vi "Avocent_build_command_OFF.vi"(8 "error in":errorcluster, 11 "Set switches":bool[](array[boolean])=[FALSE, TRUE, TRUE, FALSE, TRUE, TRUE, FALSE, FALSE, TRUE, FALSE, TRUE, TRUE, TRUE, TRUE, TRUE, TRUE, FALSE, FALSE, FALSE, FALSE, FALSE, FALSE, FALSE, FALSE, FALSE, FALSE, FALSE, FALSE, FALSE, FALSE, FALSE, FALSE] caption="Set Switches") -> (0 "error out":errorcluster, 3 "HTTP command":string="/3?3=admin,1234,1001001101000000,")   [LabVIEW 2013]
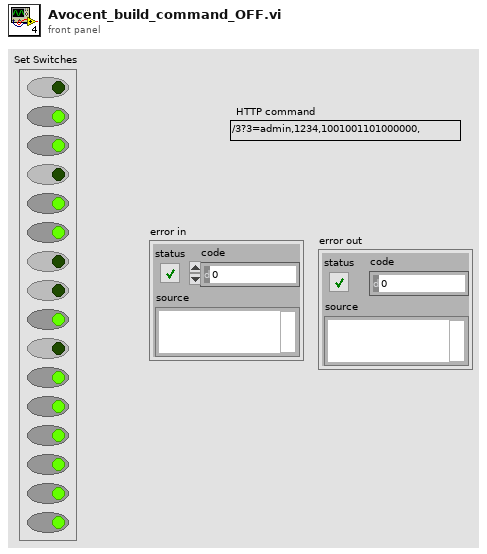
[diagram p1: front panel]
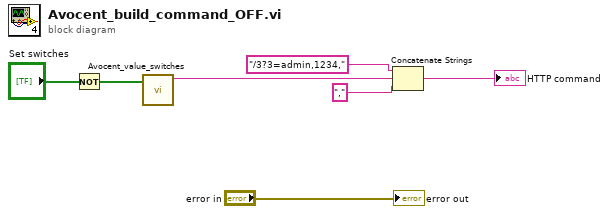
[diagram p0: block diagram]
diagram:
  n1 = Not(x="Set switches") -> (.not. x?=w1:bool[])
  n2 = call "Avocent_value_switches.vi"("Power indicator 2"=w1) -> ("spreadsheet string"=w5:string)  [unwired: 10 in]
  n3 = Concatenate Strings("/3?3=admin,1234," ("Command"), w5, "," ("Command")) -> (→"HTTP command":string)
  "error out" <- "error in"
